vi "Draw BGimg (SubVI).vi"(9 "BG Image":T1={"Path"=path "\\\\VBOXSVR\\e_drive/Repositorio MAGNIS/INF002/v0/Modules/SEQ/Mimico Display/mimico.png", "point"={"x"=0, "y"=0}}, 11 "picture in":picture) -> (3 "picture out":picture)   [LabVIEW 2014, in "SeqLoop.lvlib" / "Mimico Display.lvlib"]
uses:
  Mimico Display.lvlib
  TypeDefs/BG Image.ctl
  <vilib>/picture/picture.llb/imagedata.ctl
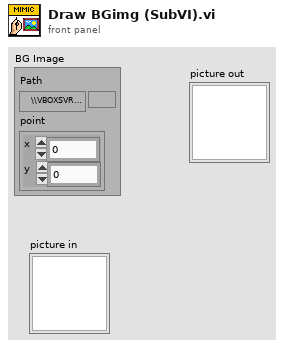
[diagram p1: front panel]
types:
  T1 = typedef "SeqLoop.lvlib/Mimico Display.lvlib/BG Image.ctl" = cluster{"Path":path, "point":cluster{"x":i16, "y":i16}}
  T2 = cluster{"left":i16, "top":i16, "right":i16, "bottom":i16}
  T3 = typedef "imagedata.ctl" = cluster{"image type":i32, "image depth":i32, "image":u8[], "mask":u8[], "colors":u32[], "Rectangle":cluster{"left":i16, "top":i16, "right":i16, "bottom":i16}}
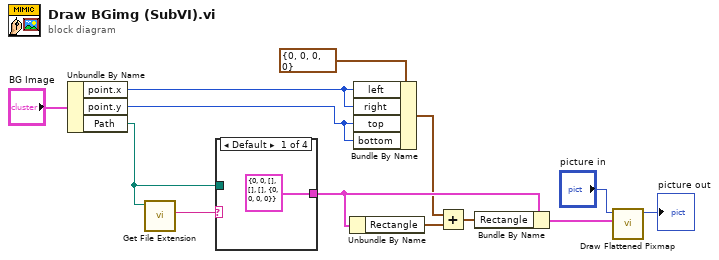
[diagram p0: block diagram]
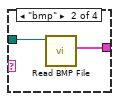
[diagram p2: hidden frame]
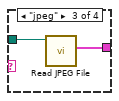
[diagram p3: hidden frame]
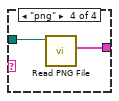
[diagram p4: hidden frame]
diagram:
  n1 = Unbundle By Name("BG Image") -> ("point.x"=w4:i16, "point.y"=w3:i16, "Path"=w2:path)
  n2 = call <vilib>:"Get File Extension.vi"("file"=w2) -> ("lowercase file extension"=w1:string)  [unwired: 7 in, 3 out]
  n3 = case shown="Default" w1 {
    tunnel: [T3 {"image type"=0, "image depth"=0, "image"=[], "mask"=[], "colors"=[], "Rectangle"={"left"=0, "top"=0, "right"=0, "bottom"=0}} ("image data") w16 w17 w19] -> w11
    tunnel: w2 -> [_ w15 w18 w20]
    frame Default {
    }
    frame "bmp" {
      n4 = call <vilib>:"Read BMP File.vi"("path to BMP file"=w15) -> ("image data"=w16:T3)  [unwired: 8 in, 2 out]
    }
    frame "jpeg" {
      n5 = call <vilib>:"Read JPEG File.vi"("path to JPEG file"=w18) -> ("image data"=w17:T3)  [unwired: 8 in, 2 out]
    }
    frame "png" {
      n6 = call <vilib>:"Read PNG File.vi"("path to PNG file"=w20) -> ("image data"=w19:T3)  [unwired: 8 in, 2 out]
    }
  }
  n7 = Unbundle By Name(w11) -> ("Rectangle"=w10:T2)
  n8 = Bundle By Name(cluster=T2 {"left"=0, "top"=0, "right"=0, "bottom"=0} ("Rectangle"), "left"=w4, "right"=w4, "top"=w3, "bottom"=w3) -> (w9:T2)
  n9 = Add(x=w9, y=w10) -> (x+y=w12:T2)
  n10 = Bundle By Name(cluster=w11, "Rectangle"=w12) -> (w13:T3)
  n11 = call <vilib>:"Draw Flattened Pixmap.vi"("image data"=w13, "picture"="picture in") -> ("new picture"=→"picture out":picture)  [unwired: 7 in]
